vi "Stop FGV.vi"(7 "Operation In":T1=enum."INIT", 8 "error in":errorcluster) -> (0 "error out":errorcluster, 2 "Stop?":bool)   [LabVIEW 2012]
doc: "This VI will check Global Stop and Errors."
uses:
  Controls/Global Stop States.ctl
  Global Stop.vi
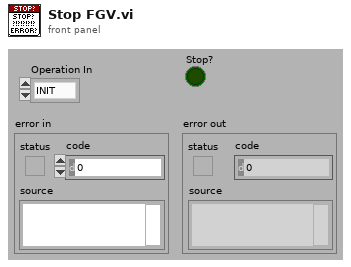
[diagram p1: front panel]
types:
  T1 = typedef "Global Stop States.ctl" = enum16{"STOP", "STATUS", "INIT"}
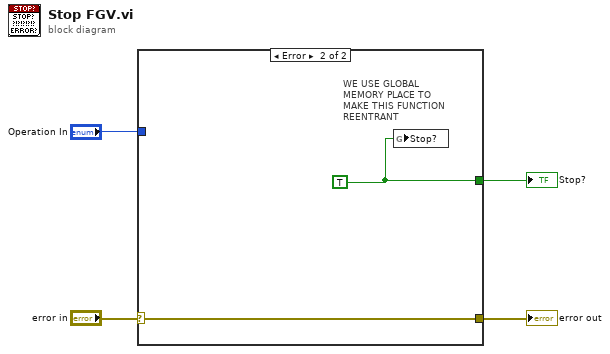
[diagram p0: block diagram]
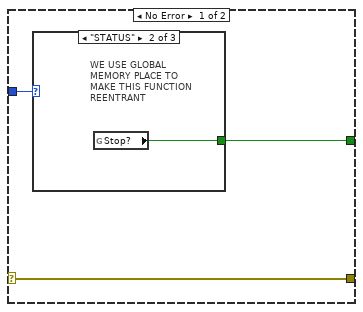
[diagram p2: hidden frame]
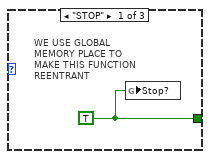
[diagram p3: hidden frame]
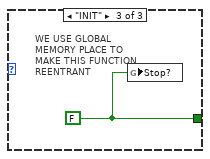
[diagram p4: hidden frame]
diagram:
  n1 = case shown="Error" "error in" {
    selector: "error in" -> [w5 w12]
    tunnel: "Operation In" -> [w7 _]
    tunnel: [w6 w11] -> w1
    tunnel: [w5 w12] -> w3
    frame No Error {
      n2 = case shown="\"STATUS\"" w7 {
        tunnel: [w8 w9 w10] -> w6
        frame "STOP" {
          w8 = TRUE ("Stop?")
          # "WE USE GLOBAL MEMORY PLACE TO MAKE THIS FUNCTION REENTRANT"
          n3 = global write "Global Stop.vi" "Stop?"(w8) -> ()
        }
        frame "STATUS" {
          # "WE USE GLOBAL MEMORY PLACE TO MAKE THIS FUNCTION REENTRANT"
          n4 = global read "Global Stop.vi" "Stop?"() -> (w9:bool)
        }
        frame "INIT" {
          w10 = FALSE ("Stop?")
          # "WE USE GLOBAL MEMORY PLACE TO MAKE THIS FUNCTION REENTRANT"
          n5 = global write "Global Stop.vi" "Stop?"(w10) -> ()
        }
      }
    }
    frame Error {
      w11 = TRUE ("Stop?")
      # "WE USE GLOBAL MEMORY PLACE TO MAKE THIS FUNCTION REENTRANT"
      n6 = global write "Global Stop.vi" "Stop?"(w11) -> ()
    }
  }
  "error out" <- w3
  "Stop?" <- w1
